vi "String_ASCII String To Data.vi"(8 "error in (no error)":errorcluster, 9 "Default":string, 11 "Value":string) -> (0 "error out":errorcluster, 3 "Data":string)   [LabVIEW 2016, in "CVT.lvlib" / "Current Value Table.lvlib"]
doc: "This VI converts data stored on disk as an ascii string into the correct data type. This VI must perform the opposite operation to the DataToASCIIString function."
uses:
  Current Value Table.lvlib
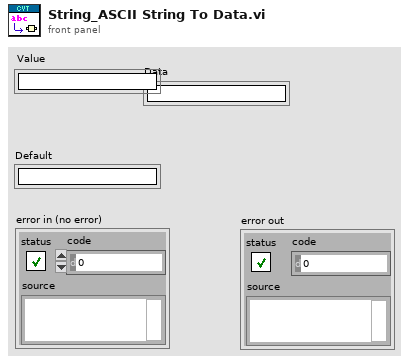
[diagram p1: front panel]
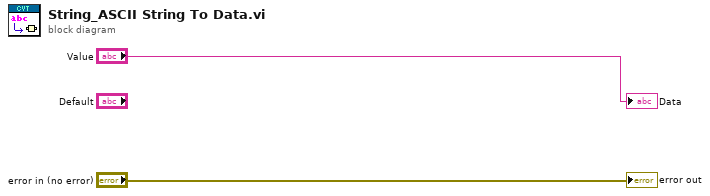
[diagram p0: block diagram]
diagram:
  "error out" <- "error in (no error)"
  "Data" <- "Value"
